vi "irrad error.vi"(8 "error in (no error)":errorcluster, 11 "Output Value":i32) -> (0 "error out":errorcluster)   [LabVIEW 2013, in "AvaSpec.lvlib" / "AVSirrad_support.lvlib"]
uses:
  AVSirrad_support.lvlib
  AvaSpec.lvlib
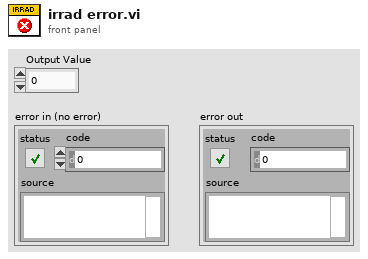
[diagram p1: front panel]
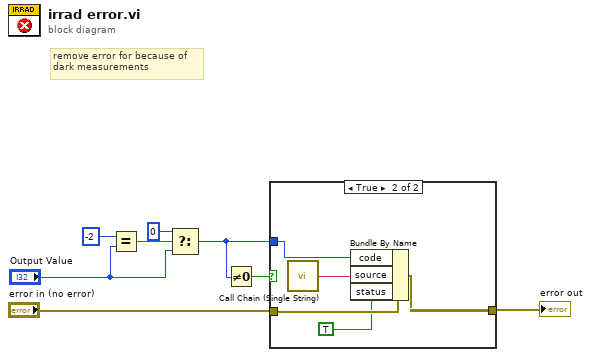
[diagram p0: block diagram]
diagram:
  # "remove error for because of \ndark measurements"
  n1 = Equal?(x=i16 -2 ("y"), y="Output Value") -> (x = y?=w5:bool)
  n2 = Select(t=i16 0, s=w5, f="Output Value") -> (s? t:f=w3:i32)
  n3 = Not Equal To 0?(x=w3) -> (x != 0?=w8:bool)
  n4 = case shown="True" w8 {
    tunnel: "error in (no error)" -> [w9 w14]
    tunnel: [w9 w13] -> w7
    tunnel: w3 -> [_ w12]
    frame False {
    }
    frame True {
      n5 = call "Call Chain (Single String).vi"() -> ("Call Chain"=w11:string)
      n6 = Bundle By Name(cluster=w14, "code"=w12, "source"=w11, "status"=TRUE) -> (w13:errorcluster)
    }
  }
  "error out" <- w7
